vi "CSMP-PostPostMsg.vi"(0 "State":string, 1 "Args":string, 2 "Source/target":string, 3 "Pre-State In":string, 4 "Pre-Args In":string, 5 "Error In":errorcluster caption="error in (no error)", 6 "Session Error":errorcluster, 8 "Module Name":string, 10 "Response Arguments":string) -> (14 "State Out":string, 15 "Args Out":string, 16 "Source/target Out":string, 17 "Pre-State Out":string, 18 "Pre-Args Out":string, 19 "Error":errorcluster)   [LabVIEW 2017, in "Communicable State Machine.lvlib"]
doc: "### CSMP-PostPostMsg.vi\n\n-- <b>Controls</b> --\n- <b>state</b>:\n- <b>args</b>:\n- <b>source/target</b>:\n- <b>Pre-State in</b>:\n- <b>Pre-Args in</b>:\n- <b>session error</b>:\n- <b>Module Name</b>:\n- <b>Response Arguments</b>:\n\n-- <b>Indicators</b> --\n- <b>state out</b>:\n- <b>args out</b>:\n- <b>source/target out</b>:\n- <b>Pre-State out</b>:\n- <b>Pre-Args out</b>:\n- <b>error</b>:"
uses:
  Communicable State Machine.lvlib
  Typedef/_Cross CSM State Data.ctl
  Typedef/_CSM_MSG_TYPE.ctl
  Typedef/_Cross CSM State Response.ctl
  Typedef/_CSM_Response Source Message.ctl
  Priority Queue/Enqueue Element.vi
  CSMQ/_CSMOFGV(lvlibp).vi
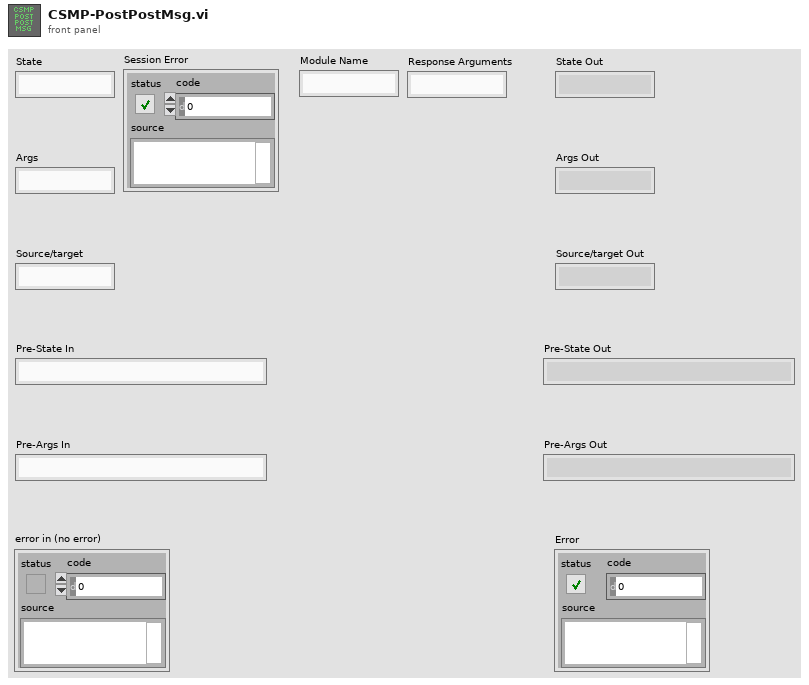
[diagram p1: front panel]
types:
  T1 = typedef "Communicable State Machine.lvlib/_CSMObj.ctl" = cluster{"info":T2, "Refs":T4}
  T2 = typedef "Communicable State Machine.lvlib/_CSMObj-Info.ctl" = cluster{"Module Name":string, "Requested Name":string, "Group Name":string, "Mode":T3, "Allowed Messages":string[]}
  T3 = typedef "Communicable State Machine.lvlib/_CSM_MODE.ctl" = enum16{"Not Exist", "Stand Alone", "CSM", "Worker", "Worker Agent", "Chain Node", "Chain"}
  T4 = typedef "Communicable State Machine.lvlib/_CSMObj-Refs.ctl" = cluster{"WatchDogQ":refnum<queue>, "CSMDataDVR":refnum<data-value>, "Queue":T5, "GroupDataDVR":refnum<data-value>, "TagMap":refnum<data-value>, "ExitEvent":refnum<user-event>, "NewStateEvent":refnum<user-event>, "StatusChangeEvent":refnum<user-event>}
  T5 = typedef "Communicable State Machine.lvlib/Priority Queue.ctl" = cluster{"HPriorityQ":refnum<queue>, "LowPriorityQ":refnum<queue>}
  T6 = typedef "Communicable State Machine.lvlib/_CSM_MSG_TYPE.ctl" = enum16{"Sync Message(-@)", "Async Message(->)", "Async without Response(->|)", "Async Response", "Broadcast(-><all>)", "Broadcast(-><status>)", "Broadcast(-><interrupt>)", "Append to JKISM States", "Append to JKISM States(High Priority)", "Broadcast(-><state>)"}
  T7 = typedef "Communicable State Machine.lvlib/_Cross CSM State Data.ctl" = cluster{"Msg Type":T6, "state":string, "args":string, "source":string, "RespQ":refnum<queue>, "Response For Message":T8, "Target":string}
  T8 = typedef "Communicable State Machine.lvlib/_CSM_Response Source Message.ctl" = cluster{"‘State":string, "’Arguments":string, "’Error":errorcluster}
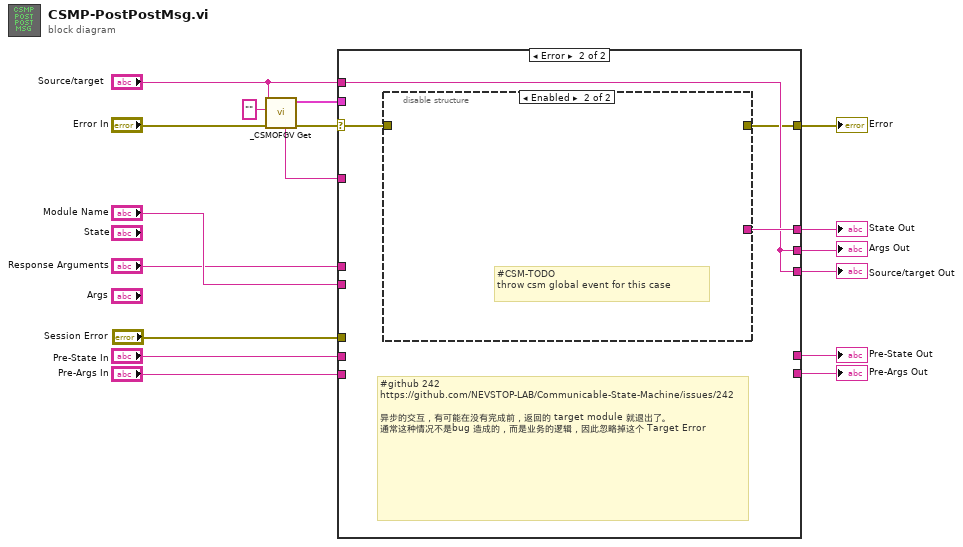
[diagram p0: block diagram]
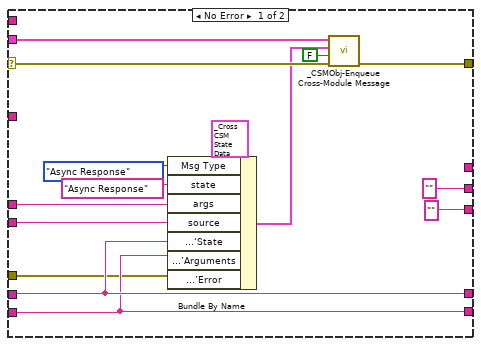
[diagram p2: hidden frame]
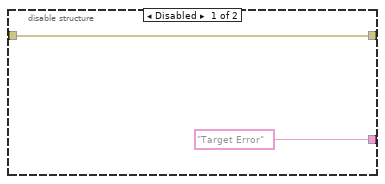
[diagram p3: hidden frame]
diagram:
  n1 = call "_CSMOFGV Get.vi"("Error In"="Error In", "Message"="", "Name (\"\" to Use UUID) In"="Source/target") -> ("error out"=w7:errorcluster, "CSM-Obj"=w8:T1, "Name"=w6:string)  [unwired: 6 in]
  n2 = case shown="Error" w7 {
    selector: w7 -> [w31 w33]
    tunnel: w8 -> [w32 _]
    tunnel: [_ w36] -> w5
    tunnel: "Source/target" -> [_ w35]
    tunnel: "Response Arguments" -> [w29 _]
    tunnel: "Module Name" -> [w28 _]
    tunnel: w6 -> [_ _]
    tunnel: [w25 _] -> w14
    tunnel: "Pre-State In" -> [w25 _]
    tunnel: "Pre-Args In" -> [w24 _]
    tunnel: [w24 _] -> w13
    tunnel: [w22 w34] -> w16
    tunnel: ["" ("Pre-State out") w35] -> w4
    tunnel: ["" ("Pre-Args out") w35] -> w3
    tunnel: "Session Error" -> [w18 _]
    frame No Error {
      n3 = Bundle By Name(cluster=T7 {"Msg Type"=enum."Sync Message(-@)", "state"="", "args"="", "source"="", "RespQ"=refnum, "Response For Message"={"‘State"="", "’Arguments"="", "’Error"={"status"=FALSE, "code"=0, "source"=""}}, "Target"=""} ("Cross JKI State Machine State"), "Msg Type"=_CSM_MSG_TYPE."Async Response", "state"="Async Response" ("Response Arguments"), "args"=w29, "source"=w28, "Response For Message.‘State"=w25, "Response For Message.’Arguments"=w24, "Response For Message.’Error"=w18) -> (w27:T7)
      n4 = call "_CSMObj-Enqueue Cross-Module Message.vi"("Error In"=w31, "High Priority? (F)"=FALSE, "Data"=w27, "CSMQ In"=w32) -> ("error out"=w22:errorcluster)  [unwired: 6 in, 1 out]
    }
    frame Error {
      # "#github 242\nhttps://github.com/NEVSTOP-LAB/Communicable-State-Machine/issues/242\n\n异步的交互，有可能在没有完成前，返回的 target module 就退出了。\n通常这种情况不是bug 造成的，而是业务的逻辑，因此忽略掉这个 Target Error"
      n5 = disable-structure shown="Enabled" {
        disable-tunnel: ["Target Error" ("before match") _] -> w36
        disable-tunnel: [w37 _] -> w34
        disable-tunnel: w33 -> [w37 _]
        frame Disabled {
        }
        frame Enabled {
          # "#CSM-TODO\nthrow csm global event for this case"
        }
      }
    }
  }
  "State Out" <- w5
  "Args Out" <- w4
  "Source/target Out" <- w3
  "Error" <- w16
  "Pre-State Out" <- w14
  "Pre-Args Out" <- w13
